vi "Sort SR List.vi"(8 "Sorting":T1(ring), 11 "list in":T2[](array[typedef]) {"Last Updated" format="%<%x>T"}) -> (3 "list out":T2[](array[typedef]) {"Last Updated" format="%<%x>T"})   [LabVIEW 2018]
uses:
  SR Cluster.ctl
  SR Status.ctl
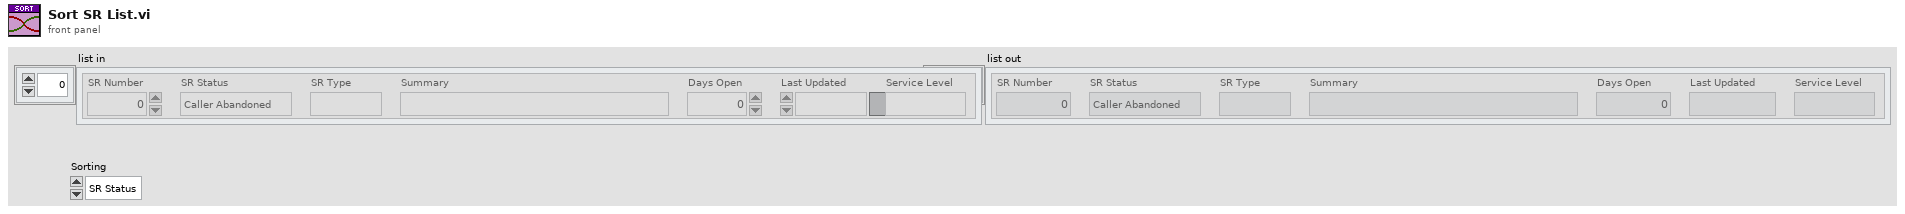
[diagram p1: front panel]
types:
  T1 = enum16{"SR Status", "Most Recent", "SR Type", "SR Number"}
  T2 = typedef "SR Cluster.ctl" = cluster{"SR Number":i32, "SR Type":string, "Summary":string, "Days Open":dbl, "Last Updated":timestamp, "Service Level":string, "SR Status":T3}
  T3 = typedef "SR Status.ctl" = enum16{"Caller Abandoned", "Created in Error", "Expired", "Forum Resolved AE", "Forum Resolved Customer", "IN WORK", "IN WORK Collab with AES", "IN WORK Collab with PSE", "IN WORK Collab with SE", "IN WORK Customer Added Note", "IN WORK Escalation", "IN WORK Wait on Customer", "Open", "Potentially Resolved", "Presumed Resolved", "RMA Approved for Return", "Resolved", "Passed Off"}
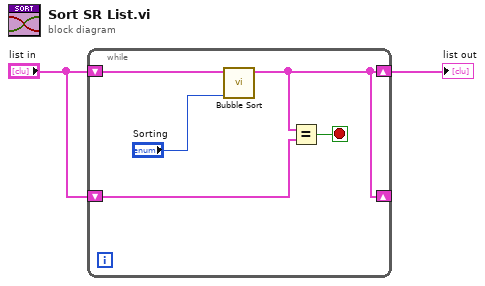
[diagram p0: block diagram]
diagram:
  n1 = while {
    shift-right: [w3] -> _
    shift-left: "list in" -> [w4]
    shift-right: [w3] -> w2
    shift-left: "list in" -> [w7]
    stop <- w5 stop-if-true
    n2 = call "Bubble Sort.vi"("Sorting"="Sorting", "list in in"=w7) -> ("list out"=w3:T2[])  [unwired: 9 in]
    n3 = Equal?(x=w3, y=w4) -> (x = y?=w5:bool)
  }
  "list out" <- w2
